vi "Xml_Save_Experiment.vi"(8 "error in (no error)":errorcluster, 10 "XML Path":path=path "D:/TEST.xml", 11 "Refnum Clust":refnum<vi>) -> (0 "error out":errorcluster, 2 "XML String Out":string)   [LabVIEW 2015]
uses:
  controls/EXPERIMENT_Inputs.ctl
  controls/LASER_Inputs.ctl
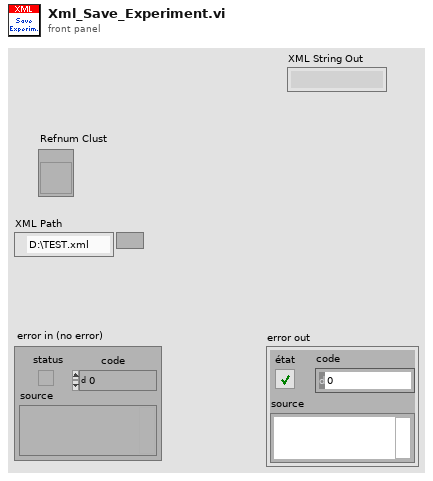
[diagram p1: front panel]
types:
  T1 = typedef "EXPERIMENT_Inputs.ctl" = cluster{"User Name":string, "Date":string, "Comment":string, "Experiment Steps":string[], "Sample Components":string[], "Molecules":string[], "Laser 1":T2, "Laser 2":T2, "Laser 3":T2}
  T2 = typedef "LASER_Inputs.ctl" = cluster{"Used":bool, "Name":string, "Reference":string, "Wavelength":dbl, "Energy":dbl}
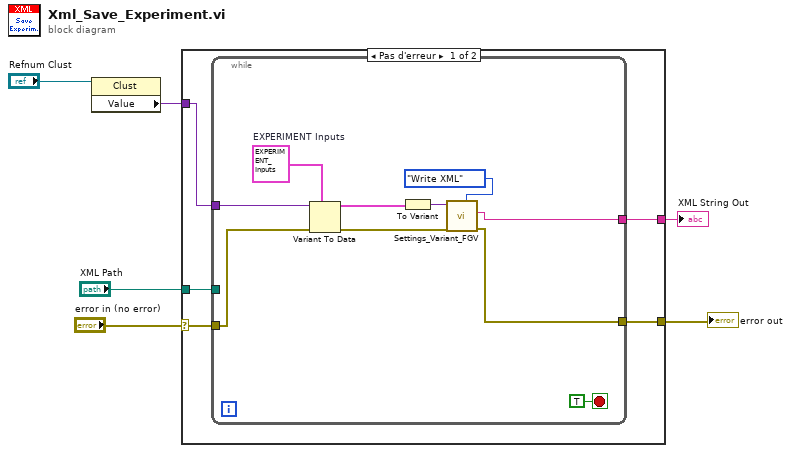
[diagram p0: block diagram]
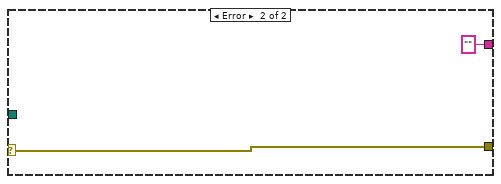
[diagram p2: hidden frame]
diagram:
  n1 = property class="Clust"(reference="Refnum Clust") -> ("Value"=w4:variant)  [unwired: 1 in, 2 out]
  n2 = case shown="Pas d'erreur" "error in (no error)" {
    selector: "error in (no error)" -> [w11 w23]
    tunnel: "XML Path" -> [w10 _]
    tunnel: w4 -> [w9 _]
    tunnel: [w8 w23] -> w3
    tunnel: [w7 "" ("XML String Out")] -> w1
    frame No Error {
      n3 = while {
        tunnel: w11 -> [w18]
        tunnel: w10 -> [_]
        tunnel: w9 -> [w17]
        tunnel: [w13] -> w8
        tunnel: [w12] -> w7
        stop <- TRUE stop-if-true
        w16 = T1 {"User Name"="", "Date"="", "Comment"="", "Experiment Steps"=[], "Sample Components"=[], "Molecules"=[], "Laser 1"={"Used"=TRUE, "Name"="Spectroscopy", "Reference"="Yag", "Wavelength"=1000.0, "Energy"=25.0}, "Laser 2"={"Used"=TRUE, "Name"="Spectroscopy", "Reference"="Yag", "Wavelength"=1000.0, "Energy"=25.0}, "Laser 3"={"Used"=TRUE, "Name"="Spectroscopy", "Reference"="Yag", "Wavelength"=1000.0, "Energy"=25.0}}  # EXPERIMENT Inputs
        n4 = Variant To Data(error in=w18, type=w16, Variant=w17) -> (data=w15:T1, error out=w14:errorcluster)
        n5 = To Variant(anything=w15) -> (Variant=w20:variant)
        n6 = call "Settings_Variant_FGV.vi"("Variant"=w20, "error in (no error)"=w14, "Command"=enum16{"Read XML", "Set", "Get", "Write XML"}."Write XML") -> ("XML String Out"=w12:string, "error out"=w13:errorcluster)  [unwired: 4 in, 1 out]
      }
    }
    frame Error {
    }
  }
  "error out" <- w3
  "XML String Out" <- w1
